vi "simulation_log_uncoupled.vi"() -> ()   [LabVIEW 2019]
uses:
  lib/libSimulationControl/libSimulationControl.lvlib
panel:
  in  "Cancel Button":bool
  out "Simulation Log":string
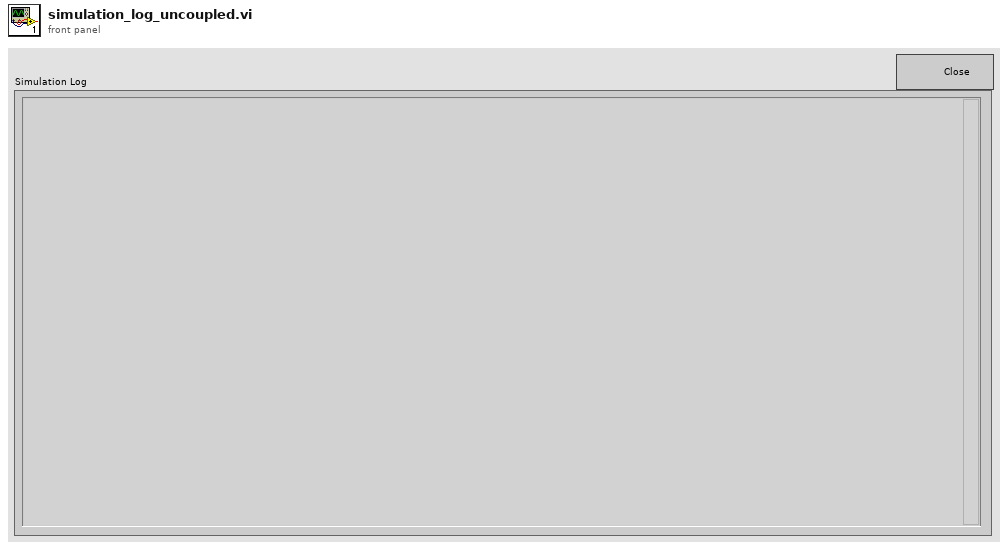
[diagram p1: front panel]
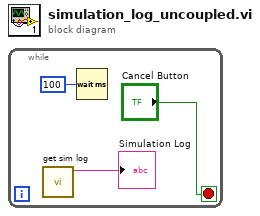
[diagram p0: block diagram]
diagram:
  n1 = while {
    stop <- "Cancel Button" stop-if-true
    n2 = call "get sim log.vi"() -> ("function return"=→"Simulation Log":string)  [unwired: 10 in, 1 out]
    n3 = Wait (ms)(milliseconds to wait=u32 100) -> ()  [unwired: 1 out]
  }
